vi "FTW-Endpoint-Bind.vi"(0 "FTW Endpoint":refnum<class "FTW-Endpoint.lvclass">, 5 "Endpoint Address":string, 7 "Requested Identity":string, 11 "error in":errorcluster) -> (4 "FTW Endpoint out":refnum<class "FTW-Endpoint.lvclass">, 6 "Actual Endpoint Address":string, 8 "Actual Identity":string, 15 "error out":errorcluster)   [LabVIEW 2013, in "FTW-Endpoint.lvclass"]
uses:
  FTW-Endpoint.lvclass
  FTW-Endpoint.lvclass/FTW-Endpoint.ctl
panel:
  # "Inputs"
  # "Outputs"
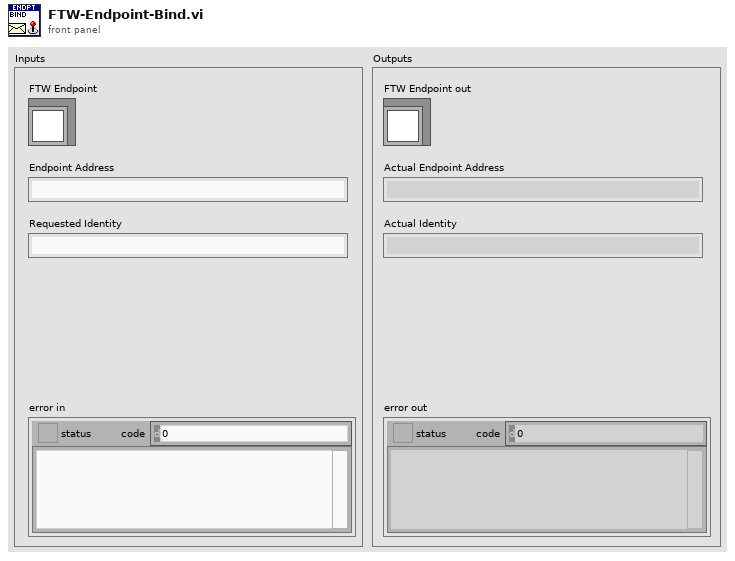
[diagram p1: front panel]
types:
  T1 = typedef "FTW-Message.ctl" = cluster{"Header":string, "Body":string, "Metadata":string}
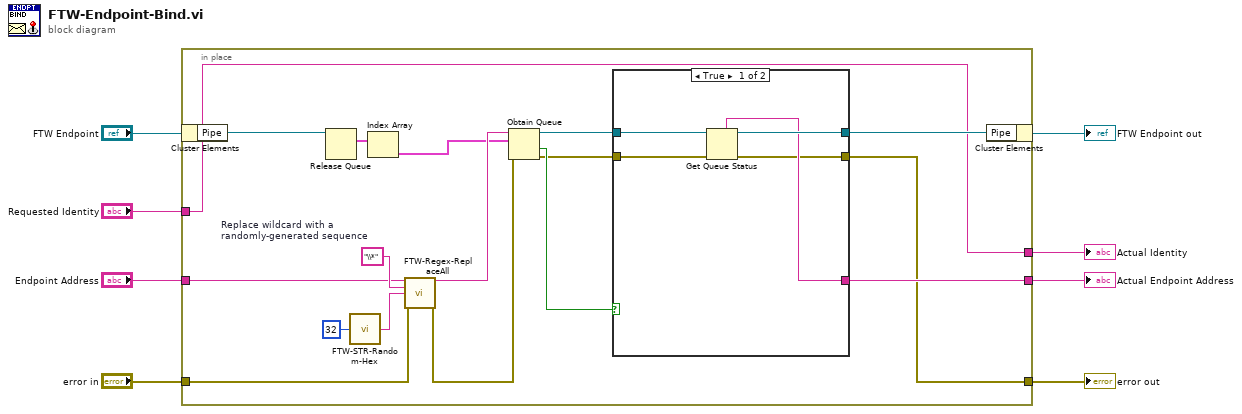
[diagram p0: block diagram]
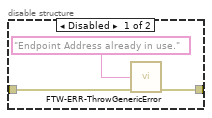
[diagram p3: hidden frame]
diagram:
  n1 = in-place {
    in-place-border: "Requested Identity" -> [w17]
    in-place-border: "error in" -> [w11]
    in-place-border: [w18] -> w8
    in-place-border: "Endpoint Address" -> [w12]
    in-place-border: [w22] -> w2
    in-place-border: [w17] -> w1
    w16 = "\\*"  # Replace wildcard with a randomly-generated sequence
    n2 = in-place-cluster #1("FTW Endpoint") -> ("Pipe"=w25:refnum<queue>)
    n3 = Release Queue(queue=w25) -> (remaining elements=w24:T1[])  [unwired: 2 in, 2 out]
    n4 = call "FTW-STR-Random-Hex.vi"("String Length"=32) -> ("Random Hex String"=w14:string)  [unwired: 3 in]
    n5 = Index Array(array=w24) -> (element=w9:T1)  [unwired: 1 in]
    n6 = call "FTW-Regex-ReplaceAll.vi"("String"=w12, "Search for (Regular Expression)"=w16, "Replace with"=w14, "error in"=w11) -> ("String out"=w13:string, "error out"=w10:errorcluster)  [unwired: 9 in, 1 out]
    n7 = Obtain Queue(name (unnamed)=w13, element data type=w9, error in (no error)=w10) -> (queue out=w20:refnum<queue>, created new?=w23:bool, error out=w19:errorcluster)  [unwired: 2 in]
    n8 = case shown="True" w23 {
      tunnel: [w27 _] -> w22
      tunnel: [w29 w32] -> w21
      tunnel: w20 -> [w30 w32]
      tunnel: w19 -> [w28 w33]
      tunnel: [w26 w31] -> w18
      frame True {
        n9 = Get Queue Status(queue=w30, error in (no error)=w28) -> (queue out=w29:refnum<queue>, queue name=w27:string, error out=w26:errorcluster)  [unwired: 1 in, 5 out]
      }
      frame False {
        n10 = disable-structure shown="Enabled" {
          disable-tunnel: w33 -> [w36 w37]
          disable-tunnel: [w35 w37] -> w31
          frame Disabled {
            n11 = call "FTW-ERR-ThrowGenericError.vi"("Error Message"="Endpoint Address already in use.", "error in"=w36) -> ("error out"=w35:errorcluster)  [unwired: 13 in]
          }
          frame Enabled {
          }
        }
      }
    }
    n12 = in-place-cluster #1("Pipe"=w21) -> (→"FTW Endpoint out":refnum<class "FTW-Endpoint.lvclass">)
  }
  "error out" <- w8
  "Actual Endpoint Address" <- w2
  "Actual Identity" <- w1
